vi "Light Color Controller.vi"(1 "Input Color":u32(colorbox), 2 "Intensity":dbl) -> (0 "Output Color":u32(colorbox))   [LabVIEW 2010]
panel:
  # "Input"
  # "Output"
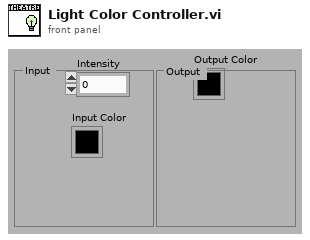
[diagram p1: front panel]
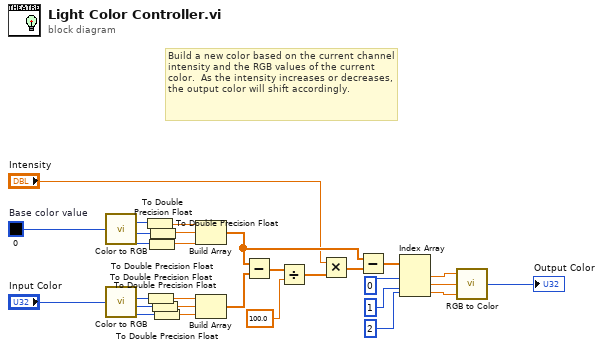
[diagram p0: block diagram]
diagram:
  w8 = u32 0  # Base color value
  # "Build a new color based on the current channel intensity and the RGB values of the current color.  As the intensity increases or decreases, the output color will shift accordingly."
  n1 = call <vilib>:"Color to RGB.vi"("Color"=w8) -> ("R"=w4:u8, "G"=w5:u8, "B"=w6:u8)  [unwired: 1 out]
  n2 = call <vilib>:"Color to RGB.vi"("Color"="Input Color") -> ("R"=w1:u8, "G"=w2:u8, "B"=w3:u8)  [unwired: 1 out]
  n3 = To Double Precision Float(number=w4) -> (double precision float=w10:dbl)
  n4 = To Double Precision Float(number=w1) -> (double precision float=w13:dbl)
  n5 = To Double Precision Float(number=w6) -> (double precision float=w12:dbl)
  n6 = To Double Precision Float(number=w5) -> (double precision float=w11:dbl)
  n7 = To Double Precision Float(number=w2) -> (double precision float=w14:dbl)
  n8 = To Double Precision Float(number=w3) -> (double precision float=w15:dbl)
  n9 = Build Array(w10, w11, w12) -> (w22:dbl[])
  n10 = Build Array(w13, w14, w15) -> (w16:dbl[])
  n11 = Subtract(x=w22, y=w16) -> (x-y=w17:dbl[])
  n12 = Divide(x=w17, y=100.0) -> (x/y=w19:dbl[])
  n13 = Multiply(x="Intensity", y=w19) -> (x*y=w21:dbl[])
  n14 = Subtract(x=w22, y=w21) -> (x-y=w23:dbl[])
  n15 = Index Array(array=w23, index #1=0, index #2=1, index #3=2) -> (element #1=w27:dbl, element #2=w28:dbl, element #3=w29:dbl)
  n16 = call <vilib>:"RGB to Color.vi"("B"=w29, "G"=w28, "R"=w27) -> ("Color"=→"Output Color":u32)
